vi "HapticSTM-write.vi"() -> ()   [LabVIEW 2017]
uses:
  SubVIs/GlobalClicksHeight.vi
  Program Files/National Instruments/LabVIEW 2019/user.lib/HapticSTM/HapticSTM.lvlib
  Program Files/National Instruments/LabVIEW 2019/user.lib/Nanonis Prog Interface V5/Nanonis Prog Interface.lvlib
panel:
  out "Safetip":bool
  out "Forces":cluster{"Fy":dbl, "Fz":dbl, "Fx":dbl} {"Fy" format="%.1f"; "Fz" format="%.1f"; "Fx" format="%.1f"}
  out "Position":cluster{"X":dbl, "Y":dbl, "Z pen":dbl, "Z":dbl}
  out "Frame Properties":cluster{"Ox":dbl, "Oy":dbl, "Fw":dbl, "Fh":dbl}
  in  "XY Write?":bool=TRUE
  in  "Z Write?":bool
  in  "Save":bool
  in  "# Sample Points":i32=4096
  in  "Depth (pA)":dbl=280.0
  in  "Shift (in)":dbl format="%.1f"
  in  "Hardness":dbl=0.7 format="%.1f"
  in  "Scaling?":u16(ring) items=["Medium", "Large", "Small"]
  out "Setpoint (pA)":dbl
  in  "Maximum (pA)":dbl=7000.0
  out "Filtered Current (pA)":dbl format="%.1f"
  out "Current (pA)":dbl format="%.1f"
  out "Z Write":dbl format="%^.1e"
  in  "Planing?":bool
  in  "Mode":u16(ring) items=["Log w/ Exp Z", "Log w/ Lin Z", "Coulomb Force", "Lennard Jones", "r^6"]
  in  "Reset Clicks":bool
  out "Clicks":i32
  in  "STOP":bool
  in  "START":bool
  # "Super Ultra Mega Haptic STM Controller 3000"
  # "Haptic Pen"
  # "Nanonis"
  # "Position"
  # "Z Controller"
  # "Force"
  # "Frame"
  # "Surface"
  # "Options"
  # "Current"
  # "No"
  # "Yes"
  # "Planing"
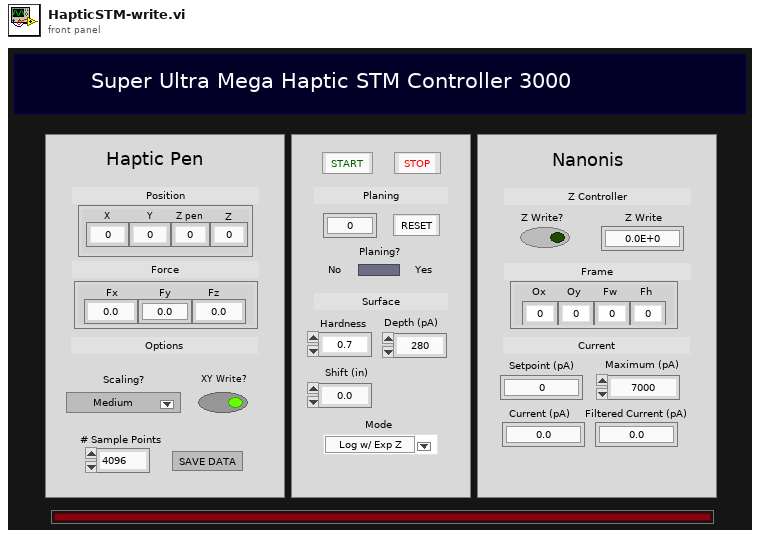
[diagram p1: front panel]
types:
  T1 = cluster{"X Origin (nm)":dbl, "Y Origin (nm)":dbl, "FW (nm)":dbl, "FH (nm)":dbl}
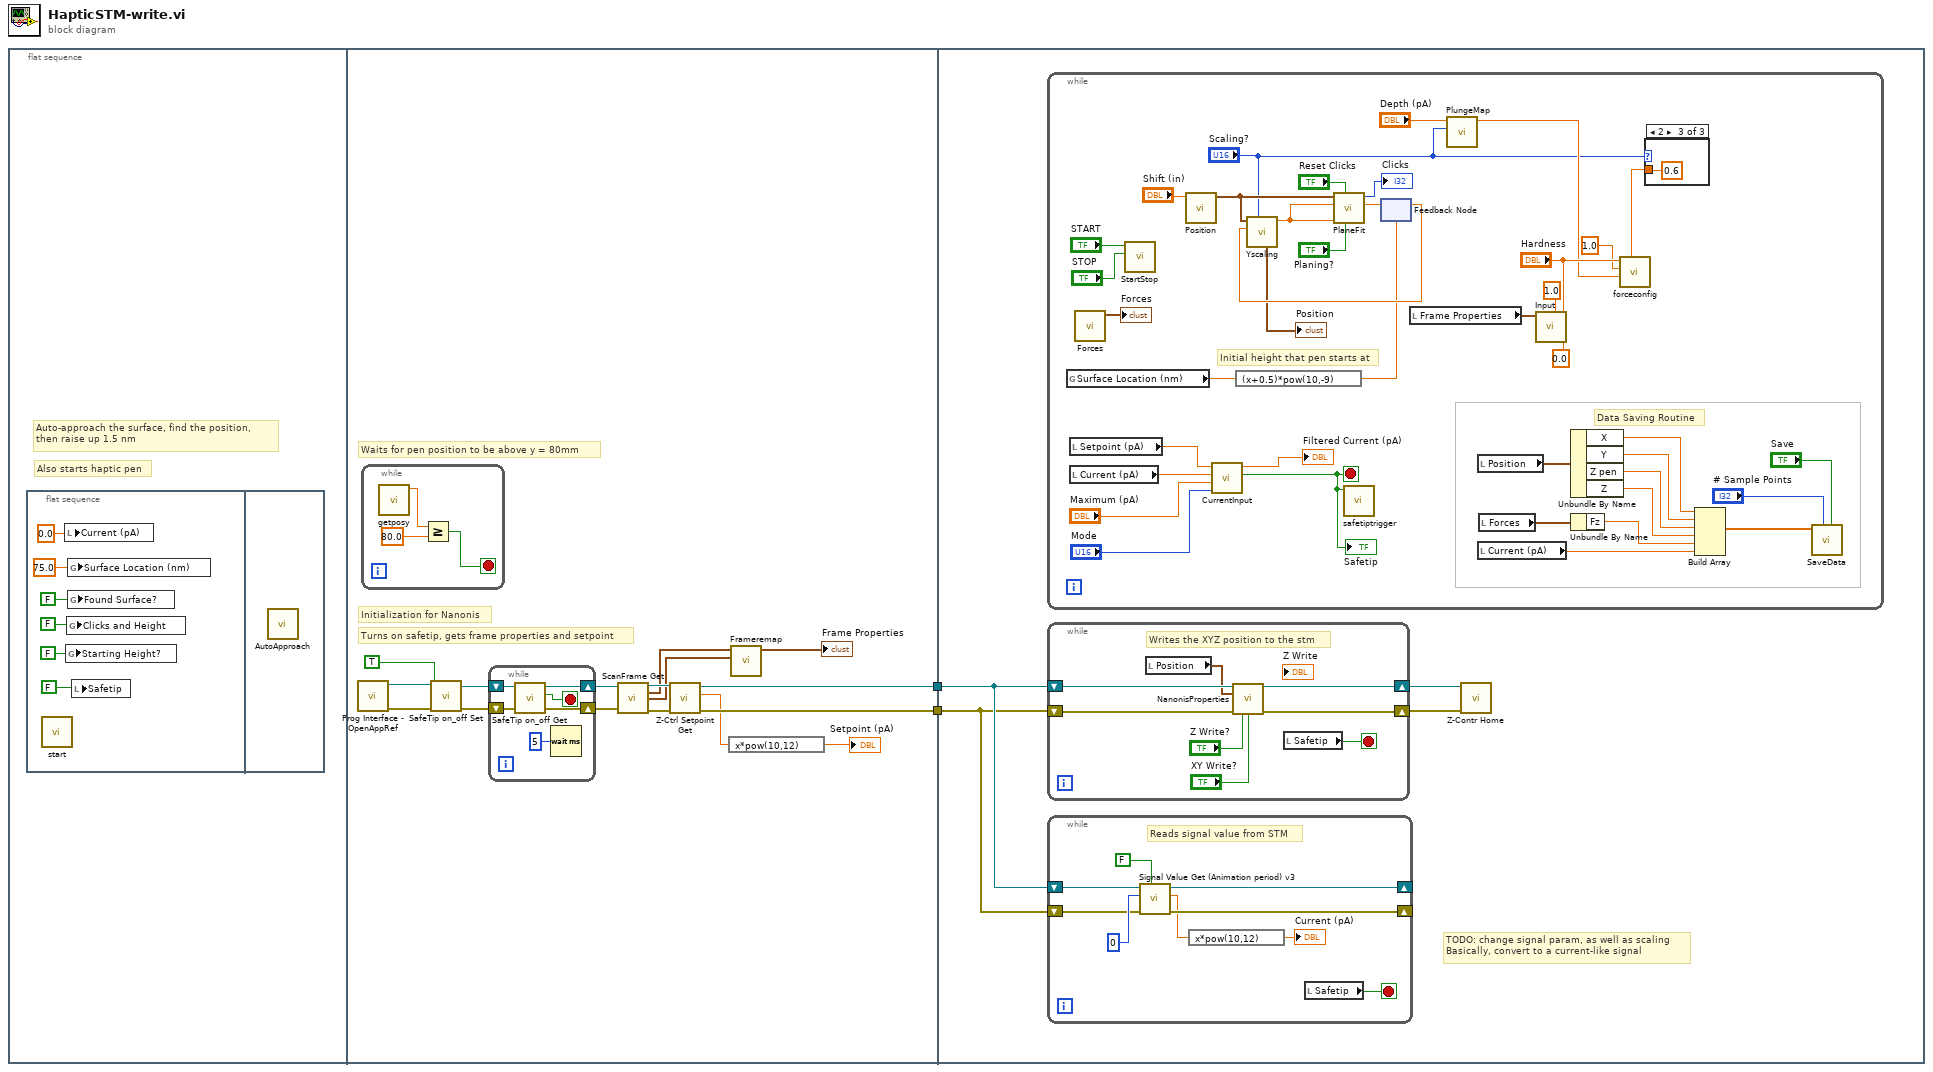
[diagram p0: block diagram]
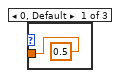
[diagram p2: hidden frame]
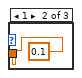
[diagram p3: hidden frame]
diagram:
  n1 = flat-sequence {
    tunnel: [w15] -> w2
    tunnel: [w14] -> w1
    tunnel: w2 -> [w37]
    tunnel: w1 -> [w36]
    frame #0 {
      # "Also starts haptic pen"
      # "Auto-approach the surface, find the position, \nthen raise up 1.5 nm"
      n2 = flat-sequence {
        frame #0 {
          n3 = call "start.vi"() -> ()  [unwired: 11 in, 1 out]
          n4 = local write "Current (pA)"(0.0 ("Current (pA)")) -> ()
          n5 = global write "GlobalClicksHeight.vi" "Starting Height?"(FALSE ("Clicks and Height")) -> ()
          n6 = global write "GlobalClicksHeight.vi" "Clicks and Height"(FALSE ("Clicks and Height")) -> ()
          n7 = global write "GlobalClicksHeight.vi" "Surface Location (nm)"(75.0 ("Surface Location")) -> ()
          n8 = global write "GlobalClicksHeight.vi" "Found Surface?"(FALSE ("Clicks and Height")) -> ()
          n9 = local write "Safetip"(FALSE ("Safe Tip?")) -> ()
        }
        frame #1 {
          n10 = call "AutoApproach.vi"() -> ()  [unwired: 12 in]
        }
      }
    }
    frame #1 {
      # "Turns on safetip, gets frame properties and setpoint"
      # "Waits for pen position to be above y = 80mm"
      # "Initialization for Nanonis"
      n11 = call <userlib>:"Prog Interface - OpenAppRef.vi"() -> ("Error out"=w18:errorcluster, "Application reference"=w17:refnum<vi>)  [unwired: 6 in]
      n12 = while {
        stop <- w25 stop-if-true
        n13 = call "getposy.vi"() -> ("function return"=w27:dbl)  [unwired: 11 in]
        n14 = Greater Or Equal?(x=w27, y=80.0) -> (x >= y?=w25:bool)
      }
      n15 = call <userlib>:"SafeTip on_off Set.vi"("error in (no error)"=w18, "SafeTip ON/OFF"=TRUE, "Application ref in"=w17) -> ("error out"=w20:errorcluster, "Application ref out"=w19:refnum<vi>)  [unwired: 7 in]
      n16 = while {
        shift-right: [w30] -> w21
        shift-left: w19 -> [w32]
        shift-right: [w29] -> w22
        shift-left: w20 -> [w31]
        stop <- w33 stop-if-true
        n17 = call <userlib>:"SafeTip on_off Get.vi"("error in (no error)"=w31, "Application ref in"=w32) -> ("error out"=w29:errorcluster, "SafeTip on/off status"=w33:bool, "Application ref out"=w30:refnum<vi>)  [unwired: 7 in]
        n18 = Wait (ms)(milliseconds to wait=u32 5) -> ()  [unwired: 1 out]
      }
      n19 = call <userlib>:"ScanFrame Get.vi"("Application ref in"=w21, "error in (no error)"=w22) -> ("Application ref out"=w23:refnum<vi>, "Center coordinates (m)"=w13:cluster{"Xc":sgl, "Yc":sgl}, "Size (m)"=w12:cluster{"Width":sgl, "Height":sgl}, "error out"=w24:errorcluster)  [unwired: 9 in, 1 out]
      n20 = call <userlib>:"Z-Ctrl Setpoint Get.vi"("error in (no error)"=w24, "Application ref in"=w23) -> ("error out"=w14:errorcluster, "Z Controller setpoint"=w10:sgl, "Application ref out"=w15:refnum<vi>)  [unwired: 6 in]
      n21 = expression code="x*pow(10,12)"(w10) -> (→"Setpoint (pA)":sgl)
      n22 = call "Frameremap.vi"("Frame Origin (m)"=w13, "Frame Size (m)"=w12) -> ("Frame Properties (Remapped)"=→"Frame Properties":T1)  [unwired: 8 in]
    }
    frame #2 {
      # "TODO: change signal param, as well as scaling\nBasically, convert to a current-like signal"
      n23 = while {
        stop <- w55 stop-if-true
        # "Data Saving Routine"
        # "Initial height that pen starts at"
        n24 = global read "GlobalClicksHeight.vi" "Surface Location (nm)"() -> (w66:dbl)
        n25 = local read "Setpoint (pA)"() -> (w64:dbl)
        n26 = local read "Current (pA)"() -> (w63:dbl)
        n27 = call "Forces.vi"() -> ("Forces"=→"Forces":cluster{"Fy":dbl, "Fz":dbl, "Fx":dbl})  [unwired: 11 in]
        n28 = call "StartStop.vi"("STOP"="STOP", "START"="START") -> ()  [unwired: 10 in]
        n29 = call "Position.vi"("Shift"="Shift (in)") -> ("Position"=w73:cluster{"X":dbl, "Y":dbl, "Zpen":dbl})  [unwired: 10 in]
        n30 = call "CurrentInput.vi"("Mode"="Mode", "Maximum (pA)"="Maximum (pA)", "Current (pA)"=w63, "Setpoint (pA)"=w64) -> ("Safetip?"=w55:bool, "Filtered Current (pA)"=→"Filtered Current (pA)":dbl)  [unwired: 6 in]
        "Safetip" <- w55
        n31 = expression code="(x+0.5)*pow(10,-9)"(w66) -> (w65:dbl)
        n32 = call "safetiptrigger.vi"("triggered"=w55) -> ()  [unwired: 11 in]
        n33 = feedback #1(w65) -> (w75:dbl)
        n34 = call "Yscaling.vi"("Scaling?"="Scaling?", "Plane Height (m)"=w75, 11:w73) -> ("y scaled (m)"=w62:dbl, "Position"=→"Position":cluster{"X":dbl, "Y":dbl, "Z pen":dbl, "Z":dbl})  [unwired: 6 in, 1 out]
        n35 = call "PlaneFit.vi"("Planing y/n?"="Planing?", "Reset Clicks"="Reset Clicks", "Y PEN"=w62, "Nano Z"=w62, "Position"=w73) -> ("Plane Height (m)"=w88:dbl, "Clicks"=→"Clicks":i32)  [unwired: 4 in, 1 out]
        n36 = feedback-in #1(w88) -> ()
        n37 = local read "Frame Properties"() -> (w74:cluster{"Ox":dbl, "Oy":dbl, "Fw":dbl, "Fh":dbl})
        n38 = call "PlungeMap.vi"("Scaling?"="Scaling?", "Input (pA)"="Depth (pA)") -> ("output"=w61:dbl)  [unwired: 9 in]
        n39 = local read "Position"() -> (w71:cluster{"X":dbl, "Y":dbl, "Z pen":dbl, "Z":dbl})
        n40 = local read "Current (pA)"() -> (w57:dbl)
        n41 = local read "Forces"() -> (w59:cluster{"Fy":dbl, "Fz":dbl, "Fx":dbl})
        n42 = call "Input.vi"("Current * 10^input"=0.0, "Sensitivity"="Hardness", "Drag"=1.0, "Frame Properties (Remapped)"=w74) -> ()  [unwired: 6 in, 2 out]
        n43 = Unbundle By Name(w71) -> ("X"=w70:dbl, "Y"=w69:dbl, "Z pen"=w68:dbl, "Z"=w67:dbl)
        n44 = Unbundle By Name(w59) -> ("Fz"=w58:dbl)
        n45 = case shown="2" "Scaling?" {
          tunnel: [0.5 0.1 0.6] -> w78
          frame 0, Default {
          }
          frame 1 {
          }
          frame 2 {
          }
        }
        n46 = call "forceconfig.vi"("spc"=w78, "c"=w61, "b"=1.0, "a"="Hardness") -> ()  [unwired: 8 in]
        n47 = Build Array(w70, w69, w68, w67, w58, w57) -> (w94:dbl[])
        n48 = call "SaveData.vi"("Save"="Save", "# Sample Points"="# Sample Points", "Data"=w94) -> ()  [unwired: 9 in]
      }
      n49 = while {
        shift-right: [w50] -> w34
        shift-left: w36 -> [w52]
        shift-right: [w51] -> w35
        shift-left: w37 -> [w53]
        stop <- w47 stop-if-true
        # "Writes the XYZ position to the stm"
        n50 = local read "Position"() -> (w48:cluster{"X":dbl, "Y":dbl, "Z pen":dbl, "Z":dbl})
        n51 = call "NanonisProperties.vi"("Application ref in"=w53, "Position"=w48, "error in (no error)"=w52, "Z Write?"="Z Write?", "XY Write?"="XY Write?") -> ("Application ref out"=w51:refnum<vi>, "error out"=w50:errorcluster)  [unwired: 9 in]
        n52 = local read "Safetip"() -> (w47:bool)
      }
      n53 = while {
        shift-right: [w43] -> _
        shift-left: w36 -> [w45]
        shift-right: [w44] -> _
        shift-left: w37 -> [w41]
        stop <- w38 stop-if-true
        # "Reads signal value from STM"
        n54 = call <userlib>:"Signal Value Get (Animation period) v3.vi"("Wait for newest data (F=False)"=FALSE, "error in (no error)"=w45, "Signal index (0-127)"=i8 0, "Application ref in"=w41) -> ("error out"=w43:errorcluster, "Signal value"=w39:sgl, "Application ref out"=w44:refnum<vi>)  [unwired: 4 in]
        n55 = expression code="x*pow(10,12)"(w39) -> (→"Current (pA)":sgl)
        n56 = local read "Safetip"() -> (w38:bool)
      }
      n57 = call <userlib>:"Z-Contr Home.vi"("Error in (no error)"=w34, "Application ref in"=w35) -> ()  [unwired: 8 in, 2 out]
    }
  }
